vi "манчестер декодер вариант 2 (SubVI).vi"(8 "Количество слов":u8, 11 "Кодированные данные":bool[](array[boolean])) -> (3 "Декодированные данные":bool[](array[boolean]))   [LabVIEW 2015]
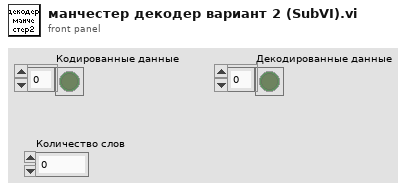
[diagram p1: front panel]
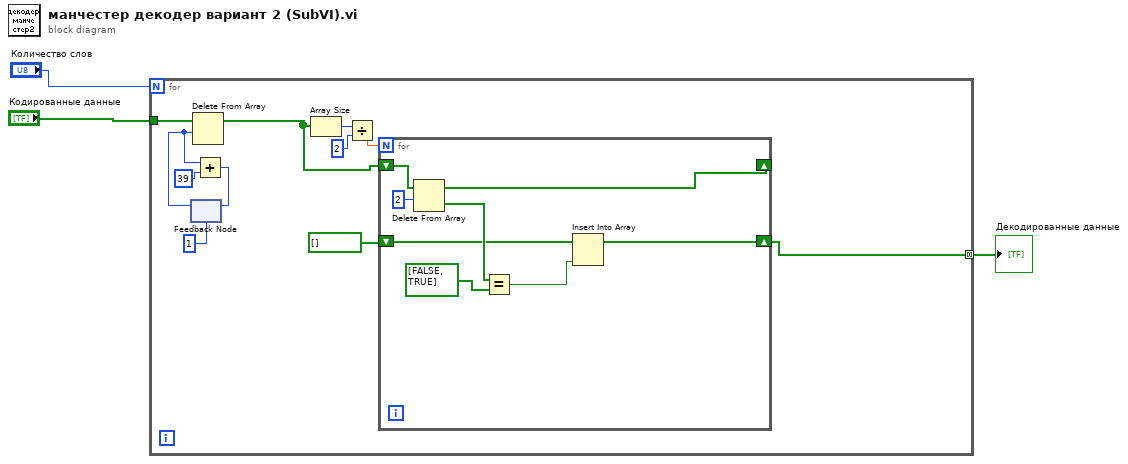
[diagram p0: block diagram]
diagram:
  n1 = for {
    N: "Количество слов" -> [_]
    tunnel: "Кодированные данные" -> [w12]
    tunnel: [w4] -> w1 mode=concatenating
    n2 = feedback #1(1 ("length")) -> (w7:i32)
    n3 = Delete From Array(array=w12, length=w7) -> (array with subset deleted=w9:bool[])  [unwired: 1 in, 1 out]
    n4 = Add(x=w7, y=39) -> (x+y=w5:i32)
    n5 = feedback-in #1(w5) -> ()
    n6 = Array Size(array=w9) -> (size(s)=w11:i32)
    n7 = Divide(x=w11, y=2) -> (x/y=w13:dbl)
    n8 = for {
      N: w13 -> [_]
      shift-right: [w20] -> _
      shift-left: w9 -> [w22]
      shift-right: [w16] -> w4
      shift-left: bool[] [] ("Array 2") -> [w17]
      n9 = Delete From Array(array=w22, length=2) -> (deleted portion=w19:bool[], array with subset deleted=w20:bool[])  [unwired: 1 in]
      n10 = Equal?(x=w19, y=bool[] [FALSE, TRUE]) -> (x = y?=w15:bool)
      n11 = Insert Into Array(array=w17, new element=w15) -> (w16:bool[])  [unwired: 1 in]
    }
  }
  "Декодированные данные" <- w1
